vi "vesselMonitoringBroadcast.vi"(0 "U":dbl[](array[numeric]), 7 "eta":dbl[](array[numeric])) -> ()   [LabVIEW 2014]
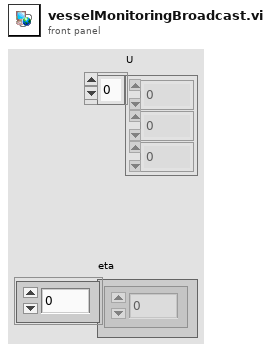
[diagram p1: front panel]
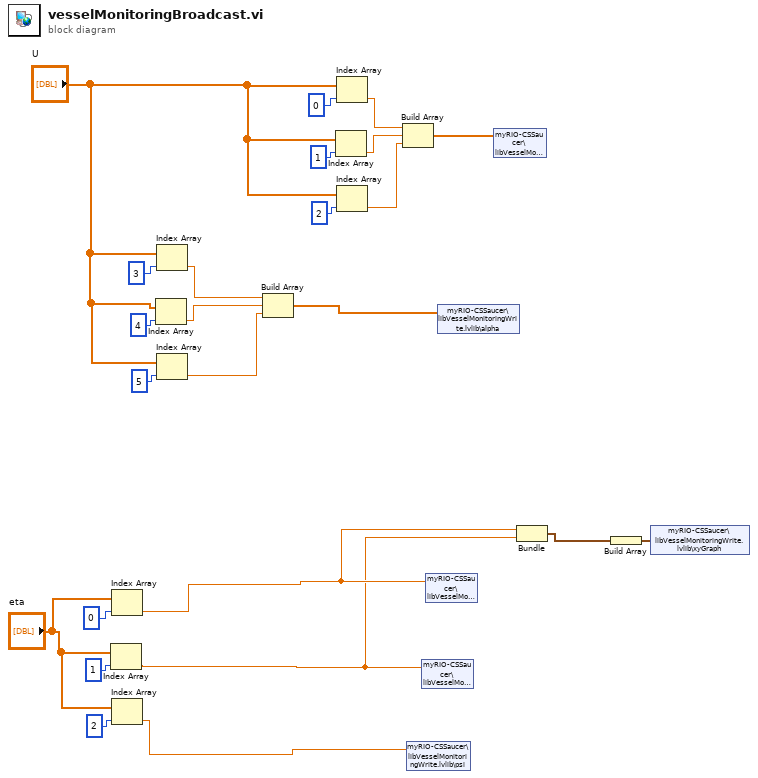
[diagram p0: block diagram]
diagram:
  n1 = Index Array(array="eta", index=1) -> (element=w2:dbl)
  n2 = Index Array(array="eta", index=0) -> (element=w3:dbl)
  n3 = Index Array(array="eta", index=2) -> (element=w1:dbl)
  n4 = Index Array(array="U", index=4) -> (element=w15:dbl)
  n5 = Index Array(array="U", index=3) -> (element=w14:dbl)
  n6 = Index Array(array="U", index=5) -> (element=w16:dbl)
  n7 = Build Array(w14, w15, w16) -> (w12:dbl[])
  n8 = Index Array(array="U", index=1) -> (element=w10:dbl)
  n9 = Index Array(array="U", index=0) -> (element=w9:dbl)
  n10 = Index Array(array="U", index=2) -> (element=w11:dbl)
  n11 = Build Array(w9, w10, w11) -> (w8:dbl[])
  n12 = shared-variable "myRIO-CSSaucer\\libVesselMonitoringWrite.lvlib\\psi"(w1) -> ()  [unwired: 1 in, 1 out]
  n13 = shared-variable "myRIO-CSSaucer\\libVesselMonitoringWrite.lvlib\\y"(w2) -> ()  [unwired: 1 in, 1 out]
  n14 = shared-variable "myRIO-CSSaucer\\libVesselMonitoringWrite.lvlib\\x"(w3) -> ()  [unwired: 1 in, 1 out]
  n15 = shared-variable "myRIO-CSSaucer\\libVesselMonitoringWrite.lvlib\\alpha"(w12) -> ()  [unwired: 1 in, 1 out]
  n16 = shared-variable "myRIO-CSSaucer\\libVesselMonitoringWrite.lvlib\\u"(w8) -> ()  [unwired: 1 in, 1 out]
  n17 = Bundle("psi"=w3, "psi"=w2) -> (w24:cluster{"psi":dbl, "psi":dbl})  [unwired: 1 in]
  n18 = Build Array(w24) -> (w23:cluster{"psi":dbl, "psi":dbl}[])
  n19 = shared-variable "myRIO-CSSaucer\\libVesselMonitoringWrite.lvlib\\xyGraph"(w23) -> ()  [unwired: 1 in, 1 out]
